vi "ReverseSolenoid.vi"(1 "Value In":u8) -> (0 "Value Out":u8)   [LabVIEW 2014]
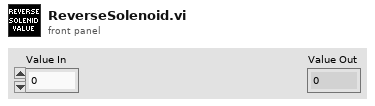
[diagram p1: front panel]
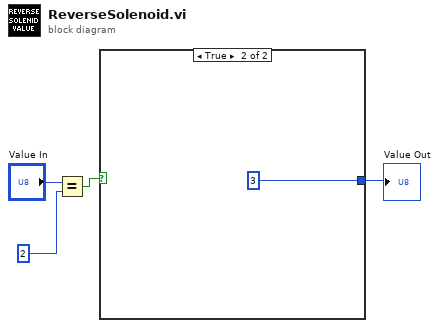
[diagram p0: block diagram]
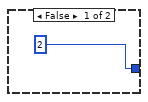
[diagram p2: hidden frame]
diagram:
  n1 = Equal?(x="Value In", y=u8 2) -> (x = y?=w4:bool)
  n2 = case shown="True" w4 {
    tunnel: [2 3] -> w1
    frame False {
    }
    frame True {
    }
  }
  "Value Out" <- w1
